vi "FGV_Timestamps_Array.vi"(0 "Action":T1=enum."Read", 5 "Size":u16, 7 "Value to add":dbl, 9 "Index":u16, 11 "error in":errorcluster) -> (4 "Timestamps_Array OUT":dbl[](array[numeric]), 15 "error out":errorcluster)   [LabVIEW 2026]
doc: "Functional Global Variable:\n- Write the value into the memory \nor\n- Read the value from the memory"
uses:
  controls/TypeDef_FGV.ctl
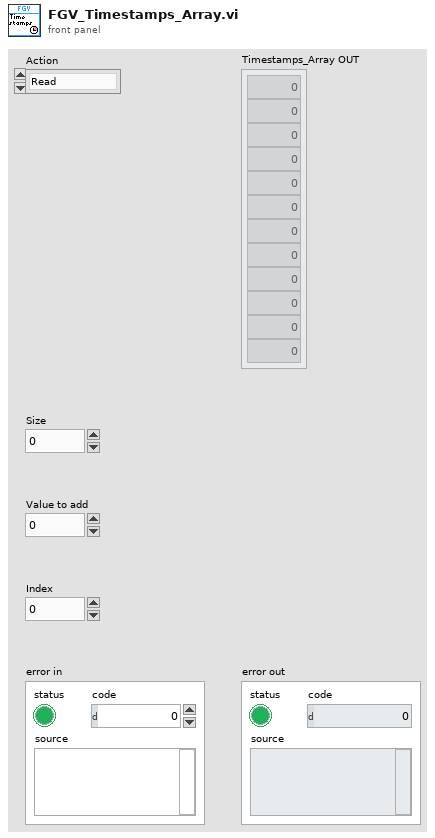
[diagram p1: front panel]
types:
  T1 = typedef "TypeDef_FGV.ctl" = enum16{"Initialize", "Add", "Read"}
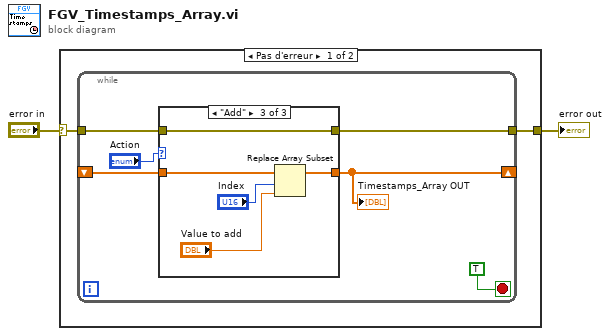
[diagram p0: block diagram]
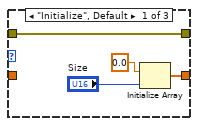
[diagram p2: hidden frame]
diagram:
  n1 = case shown="Pas d'erreur" "error in" {
    selector: "error in" -> [w4 w22]
    tunnel: [w3 w22] -> w1
    frame No Error {
      n2 = while {
        shift-right: [w7] -> _
        shift-left: _ -> [w8]
        tunnel: w4 -> [w6]
        tunnel: [w5] -> w3
        stop <- TRUE stop-if-true
        n3 = case shown="\"Add\"" "Action" {
          tunnel: w8 -> [_ w16 w20]
          tunnel: [w11 w16 w17] -> w7
          tunnel: w6 -> [w14 w15 w21]
          tunnel: [w14 w15 w21] -> w5
          frame "Initialize", Default {
            n4 = Initialize Array(0.0 ("élément"), "Size") -> (w11:dbl[])
          }
          frame "Read" {
          }
          frame "Add" {
            n5 = Replace Array Subset(array=w20, new element="Value to add", index="Index") -> (w17:dbl[])
          }
        }
        "Timestamps_Array OUT" <- w7
      }
    }
    frame Error {
    }
  }
  "error out" <- w1
